vi "AlliGator Set Calibration Type Status LEDs.vi"(8 "error in (no error)":errorcluster, 10 "Calibration Type":T1, 11 "State Indicators":refnum<vi>) -> (0 "error out":errorcluster, 1 "Message":string)   [LabVIEW 2021, in "AlliGator Phasor Calibration.lvlib"]
doc: "Sets phasor <B>Calibration Type</b> status LEDs."
uses:
  AlliGator Phasor Calibration.lvlib
  Phasor/Phasor Calibration Type.ctl
  AlliGator State Indicators List.ctl
  AlliGator Action Engine.lvlib
  AlliGator GUI.lvlib
  Phasor/Phasor.lvlib
panel:
  in  "Use Calibration Phasor Map":bool
  in  "Use Calibration Phasor Series":bool
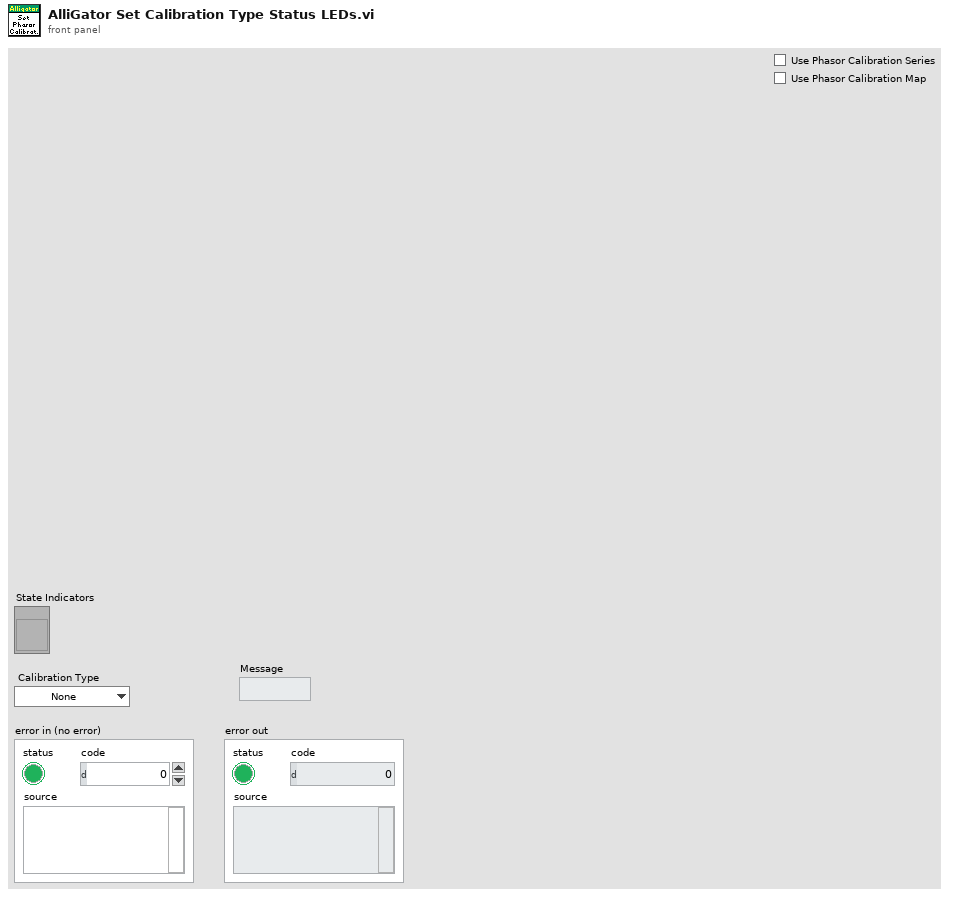
[diagram p1: front panel]
types:
  T1 = typedef "Phasor.lvlib/Phasor Calibration Type.ctl" = enum16{"None", "Single Phasor", "Phasor Series", "Phasor Map"}
  T2 = typedef "AlliGator Action Engine.lvlib/AlliGator State Indicators List.ctl" = enum16{"Phasor Calibration Defined", "Phasor Calibration Series Defined", "Phasor Calibration Map Defined", "Phasor Reference 1 Defined", "Phasor Reference 2 Defined", "Lifetime Reference 1 Defined", "Lifetime Reference 2 Defined", "Phasor Calibration Used", "Phasor Calibration Series Used", "Phasor Calibration Map Used", "Dataset Update Needed", "Phasor Plot Update Needed", "Reference/IRF Defined", "Individual IRFs Defined"}
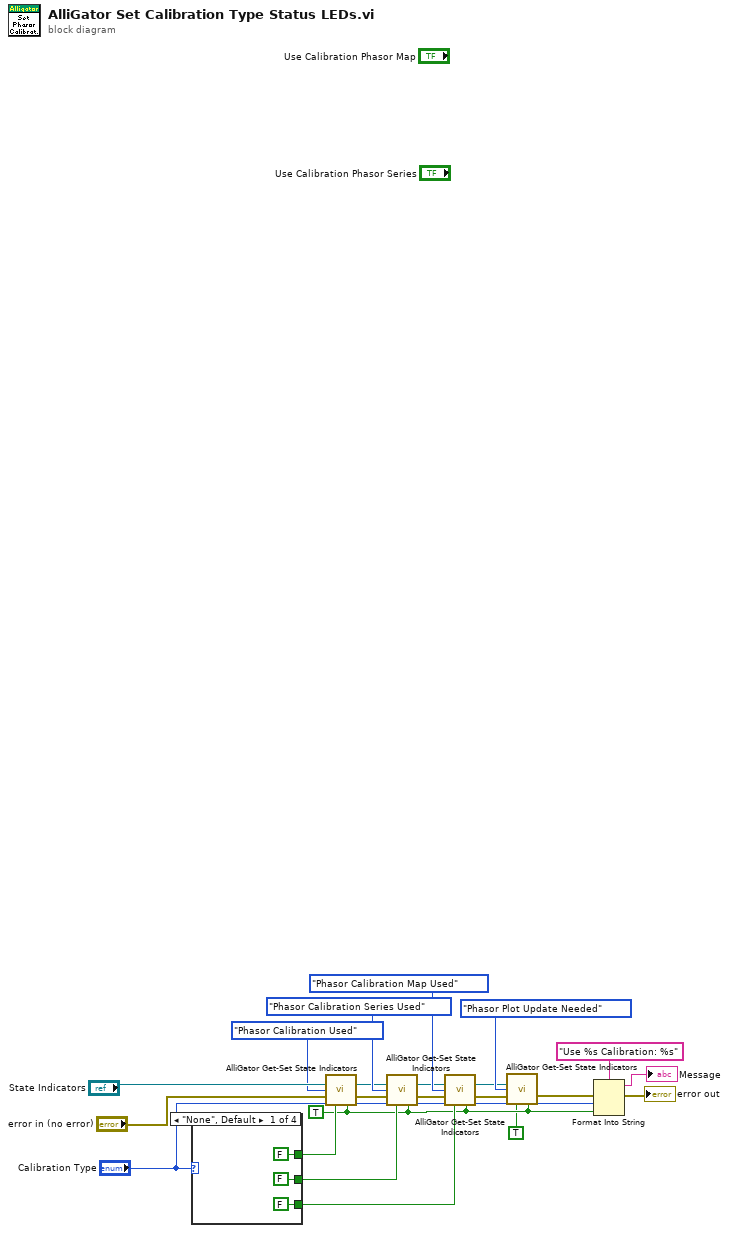
[diagram p0: block diagram]
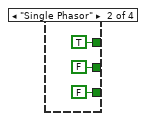
[diagram p2: hidden frame]
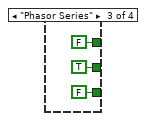
[diagram p3: hidden frame]
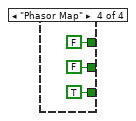
[diagram p4: hidden frame]
diagram:
  w2 = TRUE ("input 2")
  n1 = case shown="\"None\", Default" "Calibration Type" {
    tunnel: [FALSE ("ON/OFF") TRUE ("ON/OFF") FALSE ("ON/OFF") FALSE ("ON/OFF")] -> w10
    tunnel: [FALSE ("ON/OFF") FALSE ("ON/OFF") TRUE ("ON/OFF") FALSE ("ON/OFF")] -> w9
    tunnel: [FALSE ("ON/OFF") FALSE ("ON/OFF") FALSE ("ON/OFF") TRUE ("ON/OFF")] -> w8
    frame "None", Default {
    }
    frame "Single Phasor" {
    }
    frame "Phasor Series" {
    }
    frame "Phasor Map" {
    }
  }
  n2 = call "AlliGator Get-Set State Indicators.vi"("State Indicators Refnum"="State Indicators", "AlliGator State Indicators List"=AlliGator_State_Indicators_List."Phasor Calibration Used" ("Time-Gated Phasor Analysis Task List"), "Error In"="error in (no error)", "ON/OFF"=w10, "Set (T)/Get"=w2) -> ("State Indicators Refnum"=w15:refnum<vi>, "Error Out"=w14:errorcluster)  [unwired: 8 in, 1 out]
  n3 = call "AlliGator Get-Set State Indicators.vi"("State Indicators Refnum"=w15, "AlliGator State Indicators List"=AlliGator_State_Indicators_List."Phasor Calibration Series Used" ("Time-Gated Phasor Analysis Task List"), "Error In"=w14, "ON/OFF"=w9, "Set (T)/Get"=w2) -> ("State Indicators Refnum"=w13:refnum<vi>, "Error Out"=w12:errorcluster)  [unwired: 8 in, 1 out]
  n4 = call "AlliGator Get-Set State Indicators.vi"("State Indicators Refnum"=w13, "AlliGator State Indicators List"=AlliGator_State_Indicators_List."Phasor Calibration Map Used" ("Time-Gated Phasor Analysis Task List"), "Error In"=w12, "ON/OFF"=w8, "Set (T)/Get"=w2) -> ("State Indicators Refnum"=w3:refnum<vi>, "Error Out"=w6:errorcluster)  [unwired: 8 in, 1 out]
  n5 = call "AlliGator Get-Set State Indicators.vi"("State Indicators Refnum"=w3, "AlliGator State Indicators List"=AlliGator_State_Indicators_List."Phasor Plot Update Needed", "Error In"=w6, "ON/OFF"=TRUE, "Set (T)/Get"=w2) -> ("Error Out"=w5:errorcluster)  [unwired: 8 in, 2 out]
  n6 = Format Into String(format string="Use %s Calibration: %s", error in=w5, "Calibration Type", w2) -> (resulting string=→"Message":string, error out=→"error out":errorcluster)  [unwired: 1 in]
